vi "Timed Read from Hardware.vi"(8 "error in":errorcluster, 10 "Values in":dbl[](array[numeric]), 11 "Execution Unit in":refnum<class "Execution Unit.lvclass">) -> (0 "error out":errorcluster, 2 "Values out":dbl[](array[numeric]), 3 "Execution Unit out":refnum<class "Execution Unit.lvclass">)   [LabVIEW 2020, in "Ballard MIL-STD-1553 Engine.lvlib" / "Custom Device.lvlib"]
uses:
  Custom Device.lvlib
  Interfaces/Execution Unit/Execution Unit.lvclass
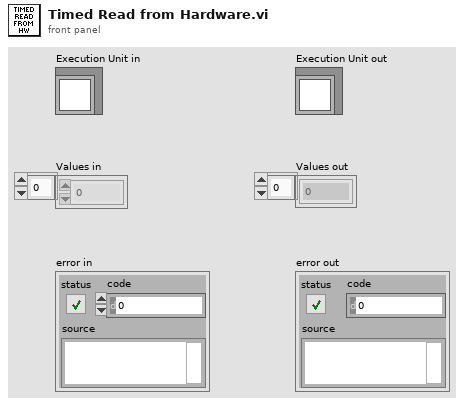
[diagram p1: front panel]
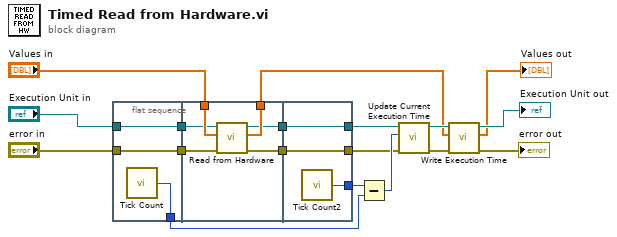
[diagram p0: block diagram]
diagram:
  n1 = flat-sequence {
    tunnel: "Execution Unit in" -> [w20]
    tunnel: "error in" -> [w21]
    tunnel: [w21] -> w15
    tunnel: [w20] -> w14
    tunnel: [w19] -> w9
    tunnel: [w27] -> w5
    tunnel: "Values in" -> [w26]
    tunnel: w15 -> [w25]
    tunnel: w14 -> [w22]
    tunnel: [w24] -> w13
    tunnel: [w23] -> w12
    tunnel: [w29] -> w3
    tunnel: [w30] -> w11
    tunnel: w13 -> [w30]
    tunnel: w12 -> [w29]
    tunnel: [w28] -> w10
    frame #0 {
      n2 = call "Tick Count"() -> ("Tick Count(uSec)"=w19:u32)
    }
    frame #1 {
      n3 = call-dynamic "Read from Hardware.vi"("error in (no error)"=w25, "Values in"=w26, "Execution Unit in"=w22) -> ("error out"=w23:errorcluster, "Values out"=w27:dbl[], "Execution Unit out"=w24:refnum<class "Execution Unit.lvclass">)  [unwired: 6 in]
    }
    frame #2 {
      n4 = call "Tick Count2"() -> ("Tick Count(uSec)"=w28:u32)
    }
  }
  n5 = Subtract(x=w10, y=w9) -> (x-y=w7:u32)
  n6 = call-dynamic "Update Current Execution Time.vi"("error in (no error)"=w3, "Current Execution Time (us)"=w7, "Execution Unit in"=w11) -> ("error out"=w2:errorcluster, "Execution Unit out"=w8:refnum<class "Execution Unit.lvclass">)  [unwired: 7 in]
  n7 = call-dynamic "Write Execution Time.vi"("error in (no error)"=w2, "Values in"=w5, "Execution Unit in"=w8) -> ("error out"=→"error out":errorcluster, "Values out"=→"Values out":dbl[], "Execution Unit out"=→"Execution Unit out":refnum<class "Execution Unit.lvclass">)  [unwired: 6 in]
